vi "Open TDMS Properties.vi"(8 "error in (no error)":errorcluster, 10 "File":path, 11 "Application Controller in":refnum<class "Application Controller.lvclass">) -> (0 "error out":errorcluster, 3 "Application Controller out":refnum<class "Application Controller.lvclass">)   [LabVIEW 2019, in "Application Controller.lvclass"]
uses:
  Application Controller.lvclass
  Plots/TDMS Properties/TDMS Properties.lvclass
  C:/GitHub/LabActor/Template Module/Template Module.lvclass
  Plots/TDMS Properties/TDMS Properties.lvclass/TDMS Properties.ctl
  <vilib>/ActorFramework/Message Enqueuer/Message Enqueuer.lvclass/Message Enqueuer.ctl
  Plots/TDMS Properties/Write File.vi
  <vilib>/ActorFramework/Message Enqueuer/Enqueue.vi
  Template Module Messages/Open Front Panel Msg/Open Front Panel Msg.lvclass
  C:/Program Files/National Instruments/LabVIEW 2019/vi.lib/ActorFramework/Message/Message.lvclass
  <vilib>/ActorFramework/Message Priority Queue/Priority Enqueue.vi
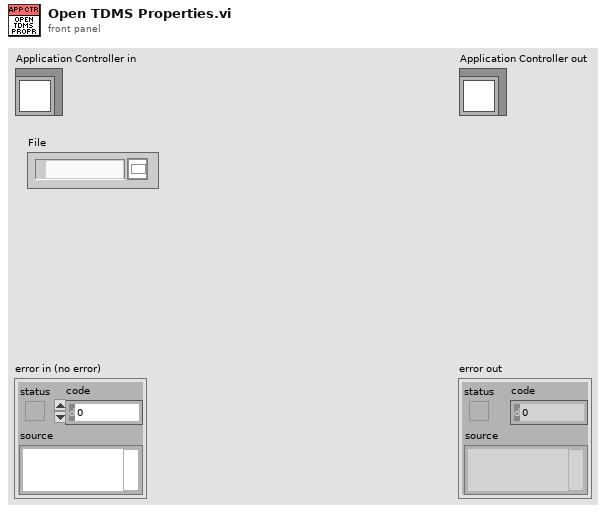
[diagram p1: front panel]
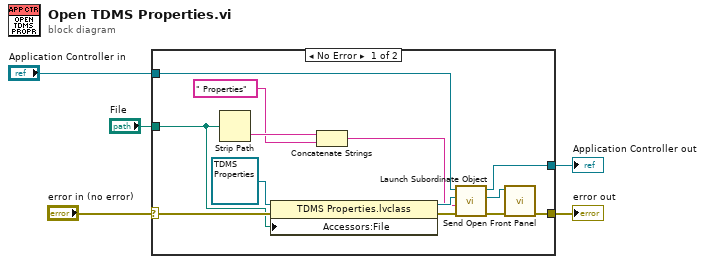
[diagram p0: block diagram]
diagram:
  n1 = case shown="No Error" "error in (no error)" {
    selector: "error in (no error)" -> [w17 w20]
    tunnel: [w8 w20] -> w4
    tunnel: [w6 w19] -> w2
    tunnel: "Application Controller in" -> [w13 w19]
    tunnel: "File" -> [w16 _]
    frame No Error {
      n2 = Strip Path(path=w16) -> (name=w15:string)  [unwired: 1 out]
      n3 = property class="TDMS Properties.lvclass"(reference=refnum<class "TDMS Properties.lvclass"> refnum ("TDMS Properties.lvclass"), error in=w17, "Accessors:File"=w16) -> (reference out=w12:refnum<class "TDMS Properties.lvclass">, error out=w7:errorcluster)
      n4 = Concatenate Strings(w15, " Properties") -> (w11:string)
      n5 = call-dynamic "Launch Subordinate Object.vi"("error in (no error)"=w7, "Name"=w11, "Subordinate Object"=w12, "Measure Object in"=w13) -> ("error out"=w10:errorcluster, "Nested Actor's Enqueuer"=w9:refnum<class "Message Enqueuer.lvclass">, "Measure Object out"=w6:refnum<class "Application Controller.lvclass">)  [unwired: 5 in]
      n6 = call "Send Open Front Panel.vi"("error in (no error)"=w10, "Message Enqueuer"=w9) -> ("error out"=w8:errorcluster)  [unwired: 8 in, 1 out]
    }
    frame Error {
    }
  }
  "error out" <- w4
  "Application Controller out" <- w2
